vi "CCE MGLD PMJD PF SubVI02.vi"(11 "captura":T2) -> (0 "orientacion correcta":bool, 1 "y":sgl, 2 "x":sgl, 3 "etiqueta detectada":bool, 5 "Image 4":T2(plugin-control))   [LabVIEW 2020]
uses:
  <vilib>/vision/Image Controls.llb/IMAQ Image.ctl
  <vilib>/vision/NI_Vision_Development_Module.lvlib
panel:
  out "Angle":sgl
  out "Number of Matches":i32
  out "Matches (real-world)":T1(array[cluster]) {"Bounding Box"."y" format="%.2f"; "Bounding Box"."x" format="%.2f"; "Score" format="%.2f"; "Scale" format="%.2f"; "Angle" format="%.2f"; "Position"."y" format="%.2f"; "Position"."x" format="%.2f"}
  out "patron":T2(plugin-control)
  out "Image 2":T2(plugin-control)
  in  "File Path":path=path "C:/Users/kitsu/Documents/SVA/proyecto final/logo.png"
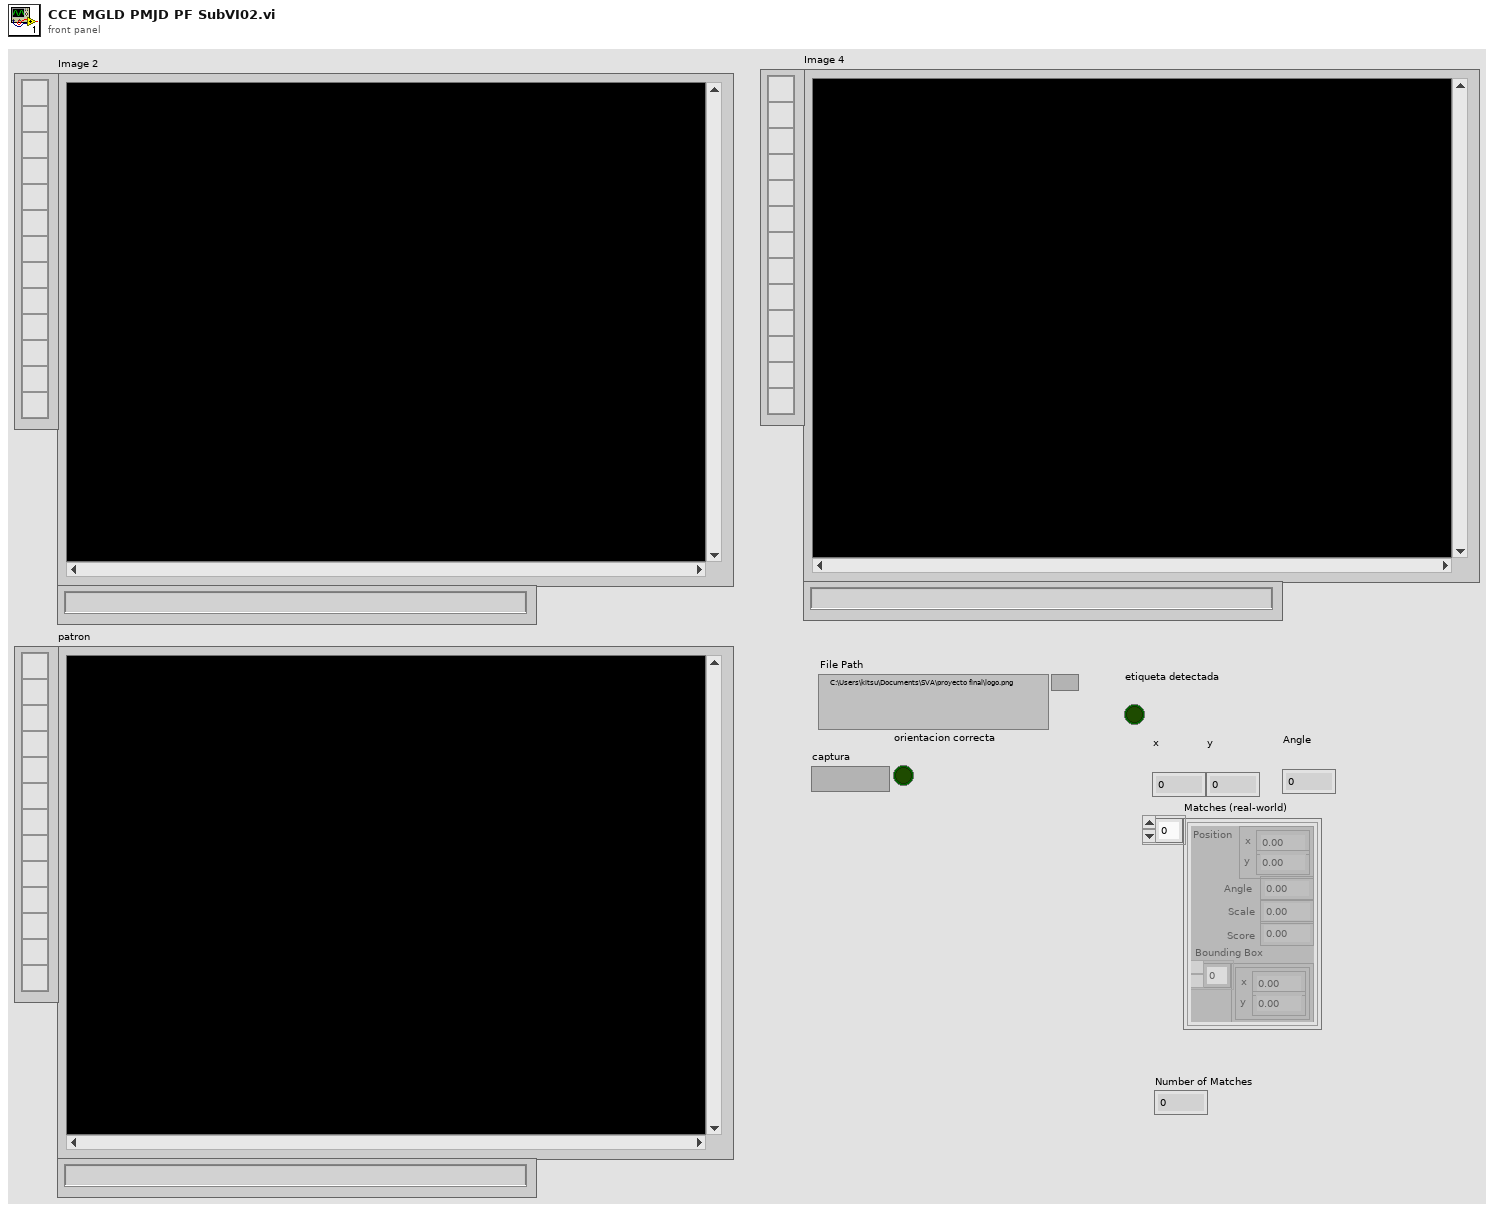
[diagram p1: front panel]
types:
  T1 = cluster{"Position":cluster{"x":sgl, "y":sgl}, "Angle":sgl, "Scale":sgl, "Score":sgl, "Bounding Box":cluster{"x":sgl, "y":sgl}[]}[]
  T2 = typedef "IMAQ Image.ctl" = refnum<image>
  T3 = cluster{"Number of Matches Requested":i32, "Minimum Match Score":sgl, "Angle Ranges":cluster{"Start Angle":sgl, "End Angle":sgl}[]}
  T4 = typedef "Image Type" = u32
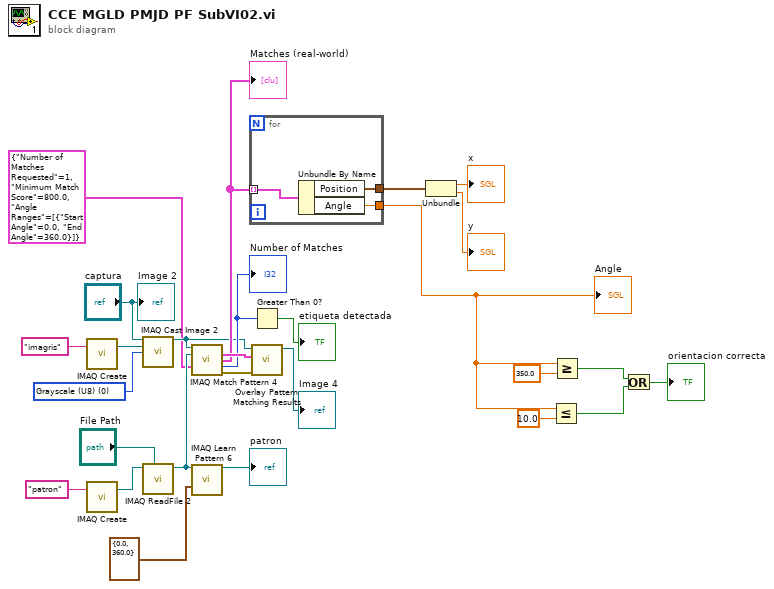
[diagram p0: block diagram]
diagram:
  w17 = T4 0 items=["Grayscale (U8)", "Grayscale (I16)", "Grayscale (SGL)", "Complex (CSG)", "RGB (U32)", "HSL (U32)", "RGB (U64)", "Grayscale (U16)"] ("Image Type")
  n1 = call "IMAQ Create"("Image Name"="imagris") -> ("New Image"=w22:T2)  [unwired: 4 in, 1 out]
  n2 = call "IMAQ Create"("Image Name"="patron") -> ("New Image"=w24:T2)  [unwired: 4 in, 1 out]
  n3 = call "IMAQ Cast Image 2"("Image Src"="captura", "Image Dst"=w22, "Image Type"=w17) -> ("Image Dst Out"=w9:T2)  [unwired: 11 in, 1 out]
  n4 = call "IMAQ ReadFile 2"("File Path"="File Path", "Image"=w24) -> ("Image Out"=w23:T2)  [unwired: 5 in, 4 out]
  n5 = call "IMAQ Match Pattern 4"("Image"=w9, "Template Image"=w23, "Parameters"=T3 {"Number of Matches Requested"=1, "Minimum Match Score"=800.0, "Angle Ranges"=[{"Start Angle"=0.0, "End Angle"=360.0}]}) -> ("Matches (pixel)"=w20:T1, "Matches (real-world)"=w16:T1, "Number of Matches"=w15:i32, "error out"=w19:errorcluster)  [unwired: 8 in, 1 out]
  "Matches (real-world)" <- w16
  "Number of Matches" <- w15
  n6 = call "IMAQ Learn Pattern 6"("Image"=w23, "Angle Range"=cluster{"Start Angle":sgl, "End Angle":sgl} {"Start Angle"=0.0, "End Angle"=360.0}) -> ("Template Image Out"=→"patron":T2)  [unwired: 11 in, 2 out]
  n7 = for {
    tunnel: w16 -> [w30] mode=indexing
    tunnel: [w29] -> w13
    tunnel: [w28] -> w6
    n8 = Unbundle By Name(w30) -> ("Position"=w29:cluster{"x":sgl, "y":sgl}, "Angle"=w28:sgl)
  }
  "Angle" <- w6
  n9 = Greater Than 0?(x=w15) -> (x > 0?=→"etiqueta detectada":bool)
  n10 = call "Overlay Pattern Matching Results.vi"("error in"=w19, "Matches"=w20, "Image"=w9) -> ("Image Out"=→"Image 4":T2)  [unwired: 7 in, 1 out]
  n11 = Unbundle(w13) -> ("x"=→"x":sgl, "y"=→"y":sgl)
  n12 = Less Or Equal?(x=w6, y=sgl 10.0) -> (x <= y?=w4:bool)
  n13 = Greater Or Equal?(x=w6, y=sgl 350.0) -> (x >= y?=w5:bool)
  n14 = Or(x=w5, y=w4) -> (x .or. y?=→"orientacion correcta":bool)
  "Image 2" <- "captura"
